vi "Log Parallel Test Retun Error.vi"(8 "code":i32, 9 "source":string, 10 "Position":u32, 11 "Parallel Test":refnum<class "Parallel Test.lvclass">) -> ()   [LabVIEW 2015, in "Parallel Test.lvclass"]
uses:
  Parallel Test.lvclass
  <vilib>/Cree, Inc/Cree Test Framework/Classes/Base Objects/Base Class/Base Class/Base Class.lvclass
  Test Class/Test Class.lvclass
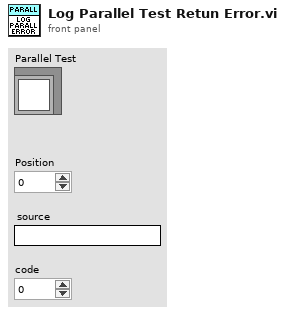
[diagram p1: front panel]
types:
  T1 = enum16{"Trace", "Debug", "Info", "Warn", "Error", "Fatal"}
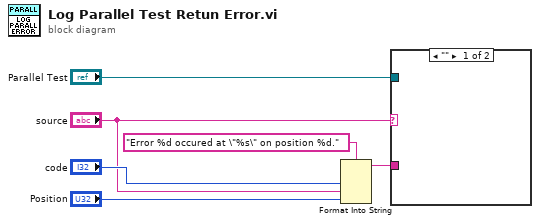
[diagram p0: block diagram]
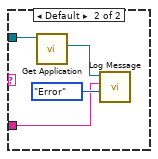
[diagram p2: hidden frame]
diagram:
  n1 = Format Into String(format string="Error %d occured at \"%s\" on position %d.", "code", "source", "Position") -> (resulting string=w2:string)  [unwired: 2 in, 1 out]
  n2 = case shown="\"\"" "source" {
    tunnel: "Parallel Test" -> [_ w9]
    tunnel: w2 -> [_ w7]
    frame "" {
    }
    frame Default {
      n3 = call "Get Application.vi"("Test Class in"=w9) -> ("Application.lvlib:Application.lvclass"=w10:refnum<class "Application.lvclass">)  [unwired: 9 in, 1 out]
      n4 = call <vilib>:"Log Message.vi"("Level"=T1."Error", "Event"=w7, "Base Class in"=w10) -> ()  [unwired: 7 in, 2 out]
    }
  }
